vi "LVIS_UpdateGlobals.vi"(8 "Error In":errorcluster, 9 "Values":string[](array[string]), 10 "Keys":string[](array[string]), 11 "Section":string) -> (0 "Error Out":errorcluster)   [LabVIEW 2015]
doc: "Loads setting file values into their respective globals."
uses:
  Globals/LVIS_DcGlobals.vi
  Globals/LVIS_IsGlobal.vi
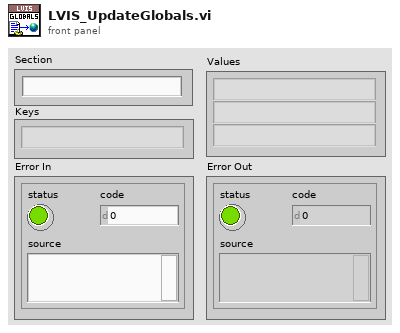
[diagram p1: front panel]
types:
  T1 = cluster{"DCIP":string, "BackupFile":string, "ErrorLog":string, "FilePosition":string}
  T2 = cluster{"PollRate":string, "ConnTimeout":string, "TxTimeout":string, "RxTimeout":string, "Port":string, "Map":string}
  T3 = cluster{"ConnTimeout":string, "TxTimeout":string, "RxTimeout":string, "Port":string, "Map":string}
  T4 = cluster{"EventName":string, "EventStart":string, "EventStop":string, "EventStatus":string, "EventClientID":string, "IS_EventID":string, "EventMeta":string, "ProductLine":string, "ProcessName":string, "Station":string, "Operator":string, "SN":string, "Model":string, "Manufacturer":string}
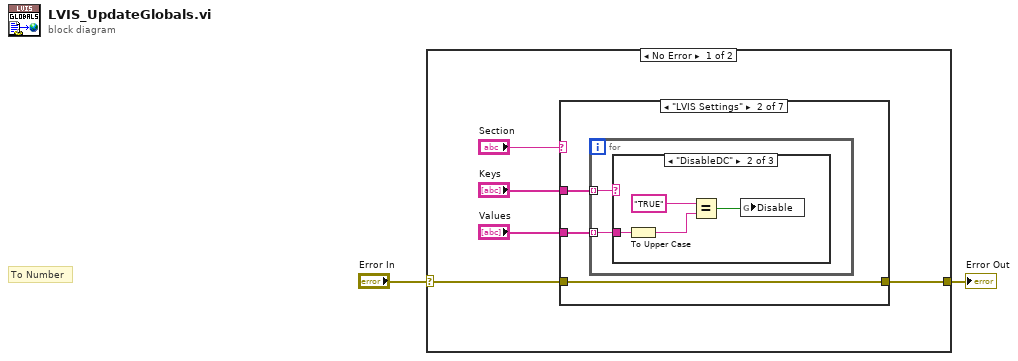
[diagram p0: block diagram]
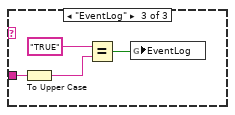
[diagram p4: hidden frame]
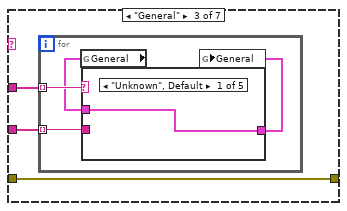
[diagram p5: hidden frame]
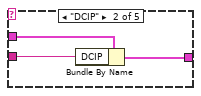
[diagram p6: hidden frame]
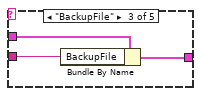
[diagram p7: hidden frame]
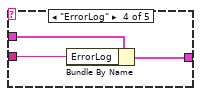
[diagram p8: hidden frame]
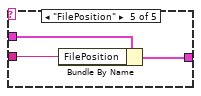
[diagram p9: hidden frame]
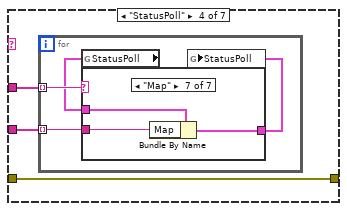
[diagram p10: hidden frame]
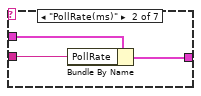
[diagram p12: hidden frame]
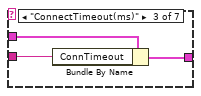
[diagram p13: hidden frame]
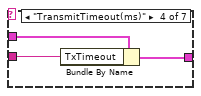
[diagram p14: hidden frame]
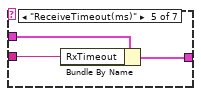
[diagram p15: hidden frame]
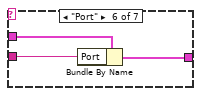
[diagram p16: hidden frame]
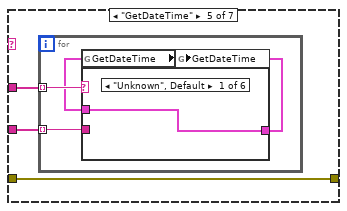
[diagram p17: hidden frame]
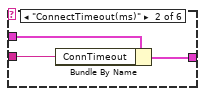
[diagram p18: hidden frame]
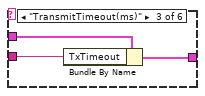
[diagram p19: hidden frame]
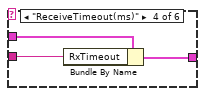
[diagram p20: hidden frame]
diagram:
  # "To Number"
  n1 = case shown="No Error" "Error In" {
    selector: "Error In" -> [w7 w164]
    tunnel: [w3 w164] -> w1
    frame No Error {
      n2 = case shown="\"LVIS Settings\"" "Section" {
        tunnel: "Values" -> [_ w10 w23 w43 w69 w92 w115]
        tunnel: w7 -> [w8 w9 w22 w42 w68 w91 w114]
        tunnel: [w8 w9 w22 w42 w68 w91 w114] -> w3
        tunnel: "Keys" -> [_ w11 w24 w44 w70 w93 w116]
        frame "Other", Default {
        }
        frame "LVIS Settings" {
          n3 = for {
            tunnel: w11 -> [w13] mode=indexing
            tunnel: w10 -> [w12] mode=indexing
            n4 = case shown="\"DisableDC\"" w13 {
              tunnel: w12 -> [_ w17 w21]
              frame "Unknown", Default {
              }
              frame "DisableDC" {
                n5 = To Upper Case(1:w17) -> (0:w16:string)
                n6 = Equal?(x="TRUE", y=w16) -> (x = y?=w14:bool)
                n7 = global write "LVIS_DcGlobals.vi" "Disable"(w14) -> ()
              }
              frame "EventLog" {
                n8 = To Upper Case(1:w21) -> (0:w20:string)
                n9 = Equal?(x="TRUE", y=w20) -> (x = y?=w18:bool)
                n10 = global write "LVIS_DcGlobals.vi" "EventLog"(w18) -> ()
              }
            }
          }
        }
        frame "General" {
          n11 = for {
            tunnel: w24 -> [w28] mode=indexing
            tunnel: w23 -> [w27] mode=indexing
            n12 = global read "LVIS_DcGlobals.vi" "General"() -> (w26:T1)
            n13 = case shown="\"Unknown\", Default" w28 {
              tunnel: w27 -> [_ w32 w35 w38 w41]
              tunnel: w26 -> [w29 w31 w34 w37 w40]
              tunnel: [w29 w30 w33 w36 w39] -> w25
              frame "Unknown", Default {
              }
              frame "DCIP" {
                n14 = Bundle By Name(cluster=w31, "DCIP"=w32) -> (w30:T1)
              }
              frame "BackupFile" {
                n15 = Bundle By Name(cluster=w34, "BackupFile"=w35) -> (w33:T1)
              }
              frame "ErrorLog" {
                n16 = Bundle By Name(cluster=w37, "ErrorLog"=w38) -> (w36:T1)
              }
              frame "FilePosition" {
                n17 = Bundle By Name(cluster=w40, "FilePosition"=w41) -> (w39:T1)
              }
            }
            n18 = global write "LVIS_DcGlobals.vi" "General"(w25) -> ()
          }
        }
        frame "StatusPoll" {
          n19 = for {
            tunnel: w44 -> [w48] mode=indexing
            tunnel: w43 -> [w47] mode=indexing
            n20 = global read "LVIS_DcGlobals.vi" "StatusPoll"() -> (w46:T2)
            n21 = case shown="\"Map\"" w48 {
              tunnel: w47 -> [_ w52 w55 w58 w61 w64 w67]
              tunnel: w46 -> [w49 w51 w54 w57 w60 w63 w66]
              tunnel: [w49 w50 w53 w56 w59 w62 w65] -> w45
              frame "Unknown", Default {
              }
              frame "PollRate(ms)" {
                n22 = Bundle By Name(cluster=w51, "PollRate"=w52) -> (w50:T2)
              }
              frame "ConnectTimeout(ms)" {
                n23 = Bundle By Name(cluster=w54, "ConnTimeout"=w55) -> (w53:T2)
              }
              frame "TransmitTimeout(ms)" {
                n24 = Bundle By Name(cluster=w57, "TxTimeout"=w58) -> (w56:T2)
              }
              frame "ReceiveTimeout(ms)" {
                n25 = Bundle By Name(cluster=w60, "RxTimeout"=w61) -> (w59:T2)
              }
              frame "Port" {
                n26 = Bundle By Name(cluster=w63, "Port"=w64) -> (w62:T2)
              }
              frame "Map" {
                n27 = Bundle By Name(cluster=w66, "Map"=w67) -> (w65:T2)
              }
            }
            n28 = global write "LVIS_DcGlobals.vi" "StatusPoll"(w45) -> ()
          }
        }
        frame "GetDateTime" {
          n29 = for {
            tunnel: w70 -> [w74] mode=indexing
            tunnel: w69 -> [w73] mode=indexing
            n30 = global read "LVIS_DcGlobals.vi" "GetDateTime"() -> (w72:T3)
            n31 = case shown="\"Unknown\", Default" w74 {
              tunnel: w73 -> [_ w78 w81 w84 w87 w90]
              tunnel: w72 -> [w75 w77 w80 w83 w86 w89]
              tunnel: [w75 w76 w79 w82 w85 w88] -> w71
              frame "Unknown", Default {
              }
              frame "ConnectTimeout(ms)" {
                n32 = Bundle By Name(cluster=w77, "ConnTimeout"=w78) -> (w76:T3)
              }
              frame "TransmitTimeout(ms)" {
                n33 = Bundle By Name(cluster=w80, "TxTimeout"=w81) -> (w79:T3)
              }
              frame "ReceiveTimeout(ms)" {
                n34 = Bundle By Name(cluster=w83, "RxTimeout"=w84) -> (w82:T3)
              }
              frame "Port" {
                n35 = Bundle By Name(cluster=w86, "Port"=w87) -> (w85:T3)
              }
              frame "Map" {
                n36 = Bundle By Name(cluster=w89, "Map"=w90) -> (w88:T3)
              }
            }
            n37 = global write "LVIS_DcGlobals.vi" "GetDateTime"(w71) -> ()
          }
        }
        frame "DataTransfer" {
          n38 = for {
            tunnel: w93 -> [w97] mode=indexing
            tunnel: w92 -> [w96] mode=indexing
            n39 = global read "LVIS_DcGlobals.vi" "DataTransfer"() -> (w95:T3)
            n40 = case shown="\"Map\"" w97 {
              tunnel: w96 -> [_ w101 w104 w107 w110 w113]
              tunnel: w95 -> [w98 w100 w103 w106 w109 w112]
              tunnel: [w98 w99 w102 w105 w108 w111] -> w94
              frame "Unknown", Default {
              }
              frame "ConnectTimeout(ms)" {
                n41 = Bundle By Name(cluster=w100, "ConnTimeout"=w101) -> (w99:T3)
              }
              frame "TransmitTimeout(ms)" {
                n42 = Bundle By Name(cluster=w103, "TxTimeout"=w104) -> (w102:T3)
              }
              frame "ReceiveTimeout(ms)" {
                n43 = Bundle By Name(cluster=w106, "RxTimeout"=w107) -> (w105:T3)
              }
              frame "Port" {
                n44 = Bundle By Name(cluster=w109, "Port"=w110) -> (w108:T3)
              }
              frame "Map" {
                n45 = Bundle By Name(cluster=w112, "Map"=w113) -> (w111:T3)
              }
            }
            n46 = global write "LVIS_DcGlobals.vi" "DataTransfer"(w94) -> ()
          }
        }
        frame "EventInfo" {
          n47 = for {
            tunnel: w116 -> [w120] mode=indexing
            tunnel: w115 -> [w119] mode=indexing
            n48 = global read "LVIS_IsGlobal.vi" "EventInfo"() -> (w118:T4)
            n49 = case shown="\"Manufacturer\"" w120 {
              tunnel: w119 -> [_ w124 w127 w130 w133 w136 w139 w142 w145 w148 w151 w154 w157 w160 w163]
              tunnel: w118 -> [w121 w123 w126 w129 w132 w135 w138 w141 w144 w147 w150 w153 w156 w159 w162]
              tunnel: [w121 w122 w125 w128 w131 w134 w137 w140 w143 w146 w149 w152 w155 w158 w161] -> w117
              frame "Unknown", Default {
              }
              frame "EventName" {
                n50 = Bundle By Name(cluster=w123, "EventName"=w124) -> (w122:T4)
              }
              frame "EventStart" {
                n51 = Bundle By Name(cluster=w126, "EventStart"=w127) -> (w125:T4)
              }
              frame "EventStop" {
                n52 = Bundle By Name(cluster=w129, "EventStop"=w130) -> (w128:T4)
              }
              frame "EventStatus" {
                n53 = Bundle By Name(cluster=w132, "EventStatus"=w133) -> (w131:T4)
              }
              frame "EventClientID" {
                n54 = Bundle By Name(cluster=w135, "EventClientID"=w136) -> (w134:T4)
              }
              frame "IS_EventID" {
                n55 = Bundle By Name(cluster=w138, "IS_EventID"=w139) -> (w137:T4)
              }
              frame "EventMeta" {
                n56 = Bundle By Name(cluster=w141, "EventMeta"=w142) -> (w140:T4)
              }
              frame "ProductLine" {
                n57 = Bundle By Name(cluster=w144, "ProductLine"=w145) -> (w143:T4)
              }
              frame "ProcessName" {
                n58 = Bundle By Name(cluster=w147, "ProcessName"=w148) -> (w146:T4)
              }
              frame "Station" {
                n59 = Bundle By Name(cluster=w150, "Station"=w151) -> (w149:T4)
              }
              frame "Operator" {
                n60 = Bundle By Name(cluster=w153, "Operator"=w154) -> (w152:T4)
              }
              frame "SN" {
                n61 = Bundle By Name(cluster=w156, "SN"=w157) -> (w155:T4)
              }
              frame "Model" {
                n62 = Bundle By Name(cluster=w159, "Model"=w160) -> (w158:T4)
              }
              frame "Manufacturer" {
                n63 = Bundle By Name(cluster=w162, "Model"=w163) -> (w161:T4)
              }
            }
            n64 = global write "LVIS_IsGlobal.vi" "EventInfo"(w117) -> ()
          }
        }
      }
    }
    frame Error {
    }
  }
  "Error Out" <- w1
